vi "quiz 3.4.vi"() -> ()   [LabVIEW 2017]
panel:
  out "Tab Control":T1(tab)
  in  "Ingresar":bool
  in  "usuario":string
  in  "Contraseña":string
  in  "eliminar":bool
  in  "agregar":bool
  in  "Lista":bool
  in  "FINALIZAR":bool
  in  "Volver":bool
  in  "AÑADIR":bool
  in  "contraseña":string
  in  "usuario":string
  in  "Quitar":bool
  in  "usuario a eliminar":string
  in  "FINALIZAR 3":bool
  in  "Volver 2":bool
  out "Seccion Inicada por:":string
  in  "FINALIZAR 2":bool
  in  "FINALIZAR 4":bool
  in  "Volver 3":bool
  out "USUARIOS":string
  # "¿QUE DESEA REALIZAR?"
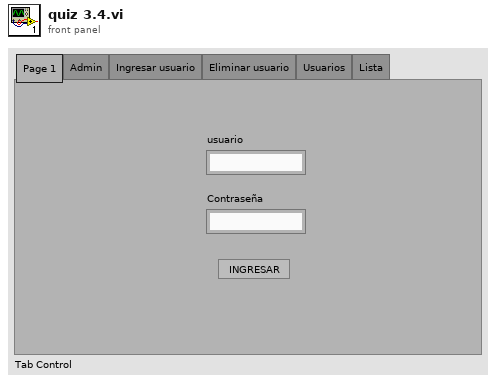
[diagram p1: front panel]
types:
  T1 = enum32{"Page 1", "Admin", "Ingresar usuario", "Eliminar usuario", "Usuarios", "Lista"}
  T2 = enum16{"open", "replace", "create", "open or create", "replace or create", "replace or create with confirmation"}
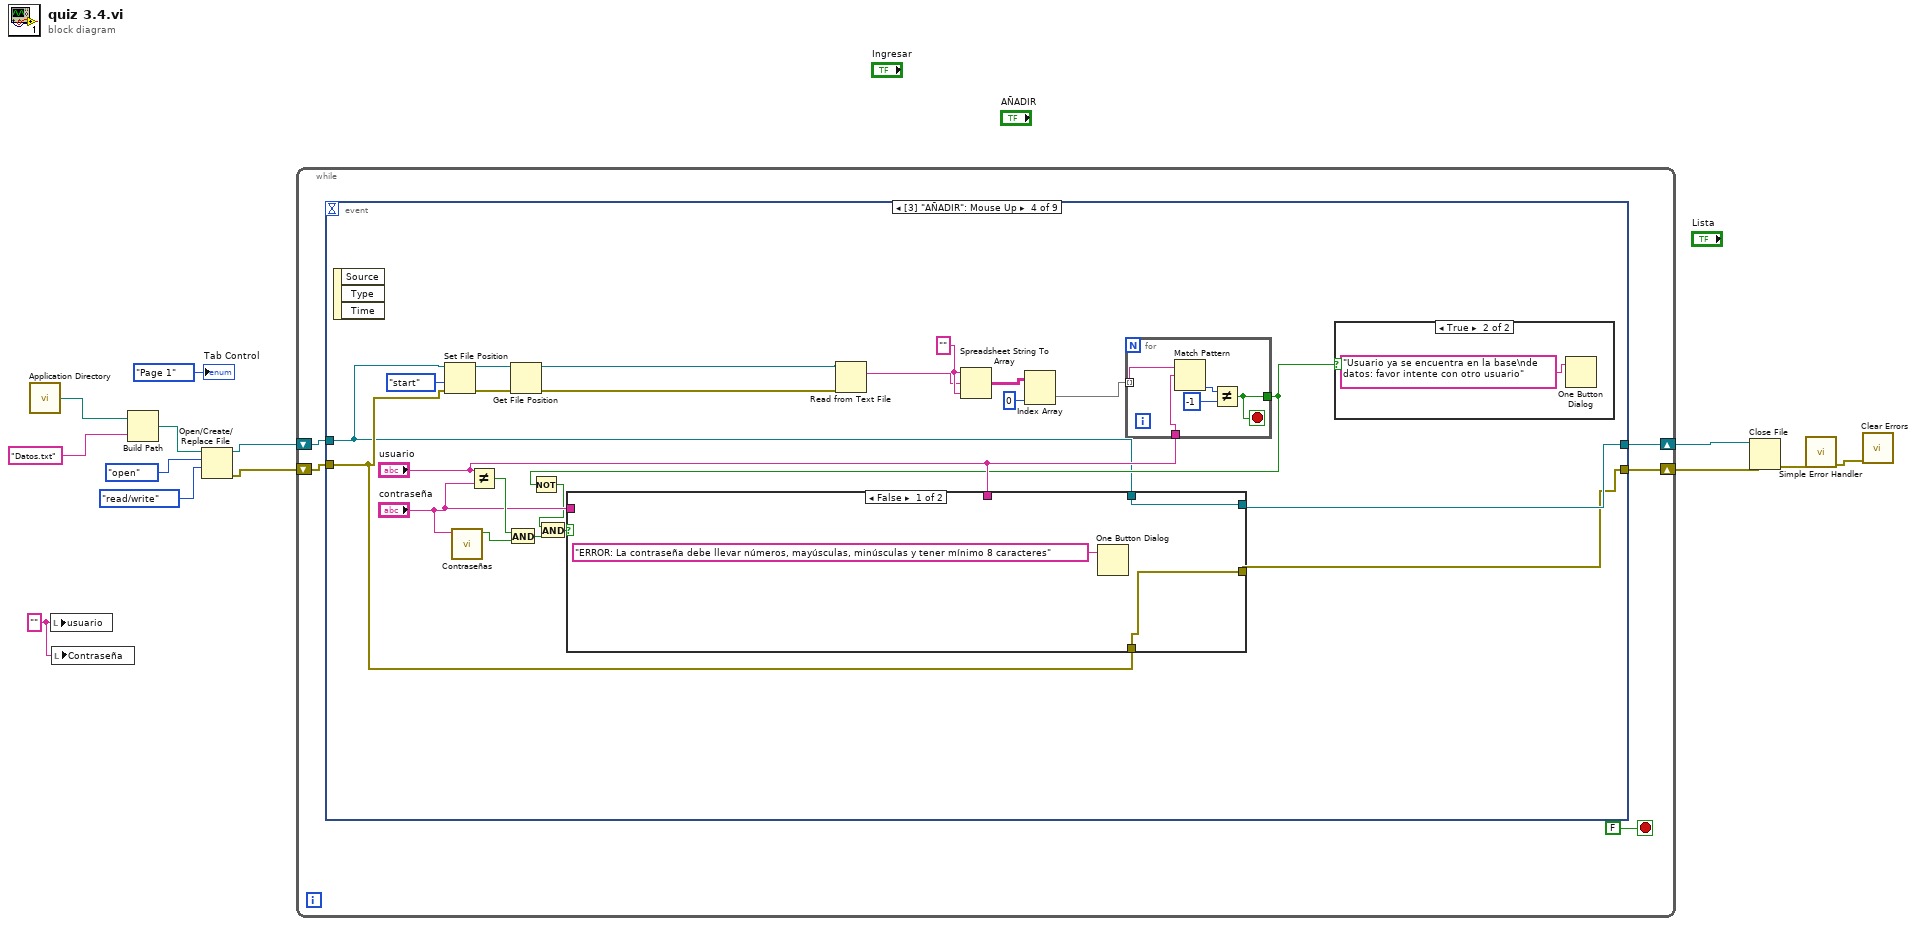
[diagram p0: block diagram]
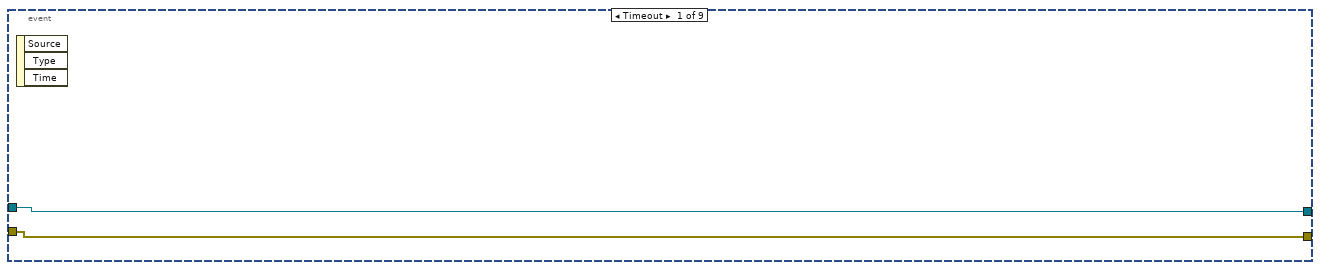
[diagram p2: hidden frame]
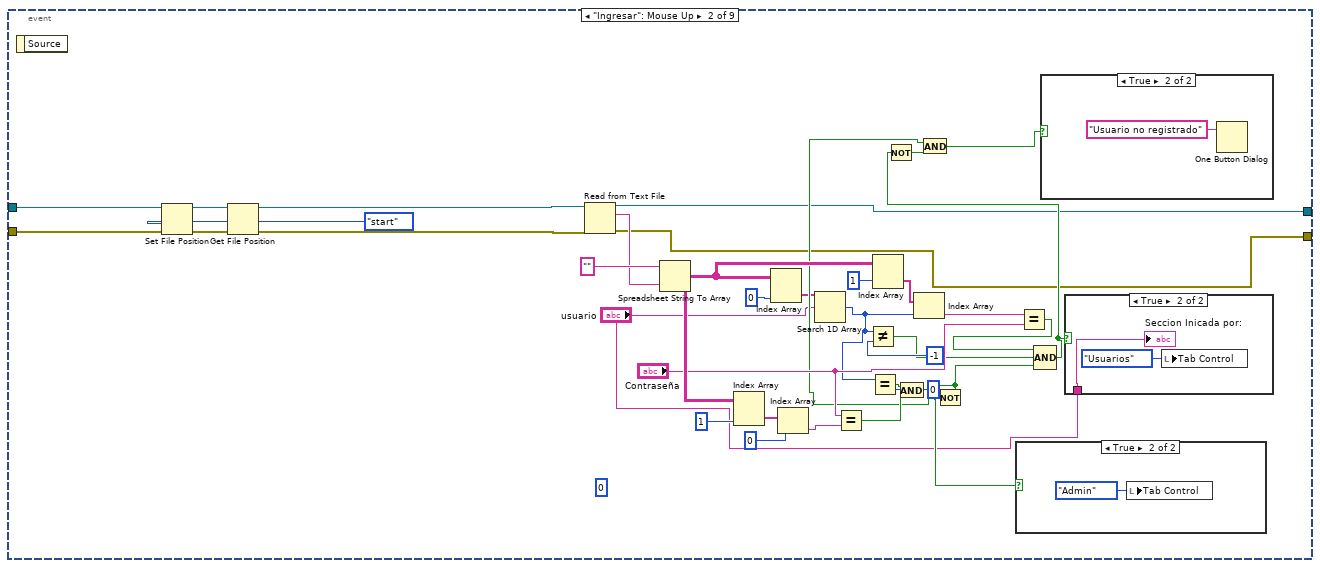
[diagram p3: hidden frame]
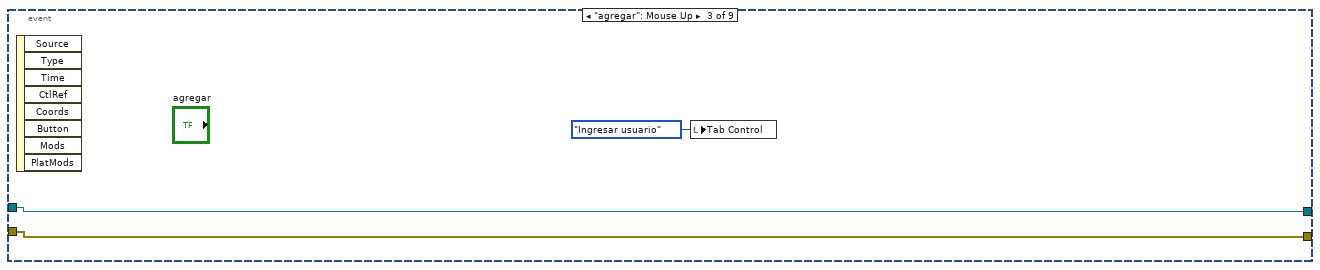
[diagram p7: hidden frame]
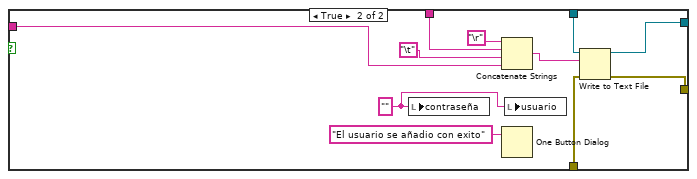
[diagram p9: hidden frame]
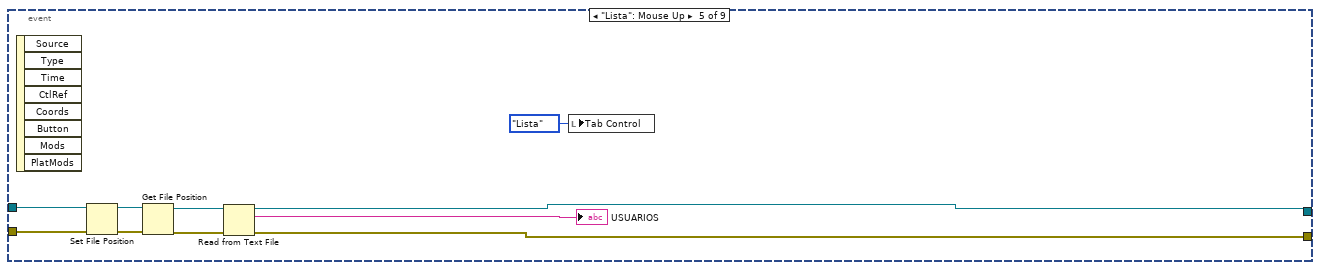
[diagram p10: hidden frame]
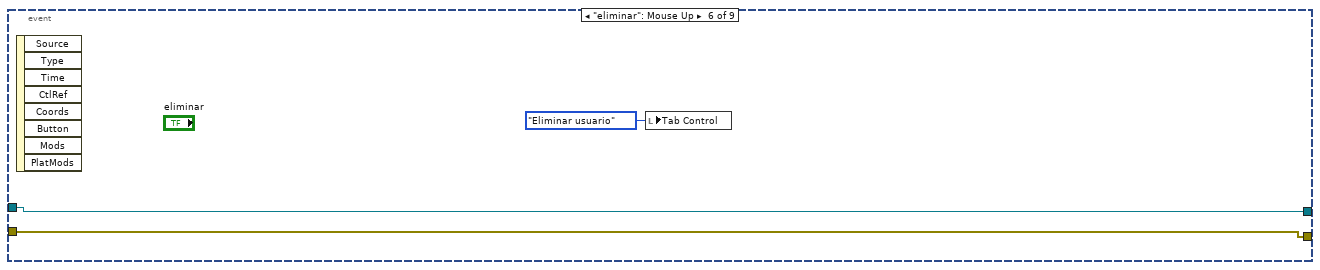
[diagram p11: hidden frame]
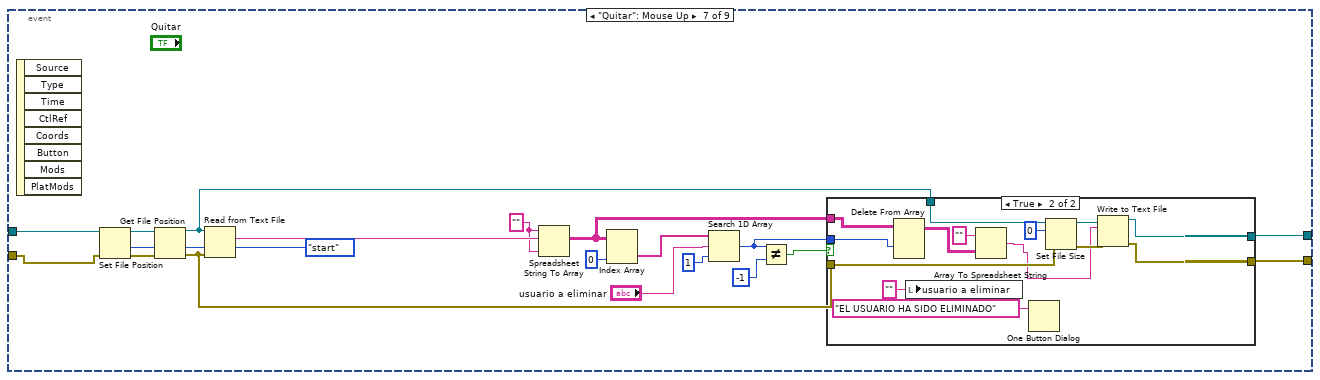
[diagram p12: hidden frame]
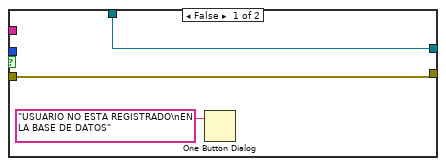
[diagram p13: hidden frame]
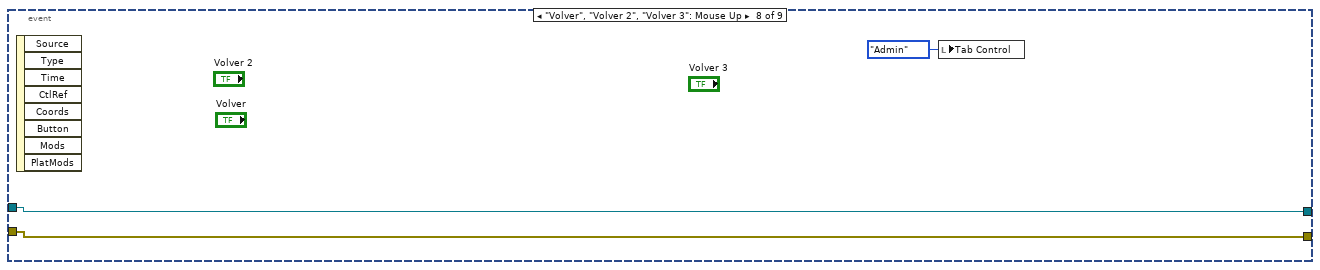
[diagram p14: hidden frame]
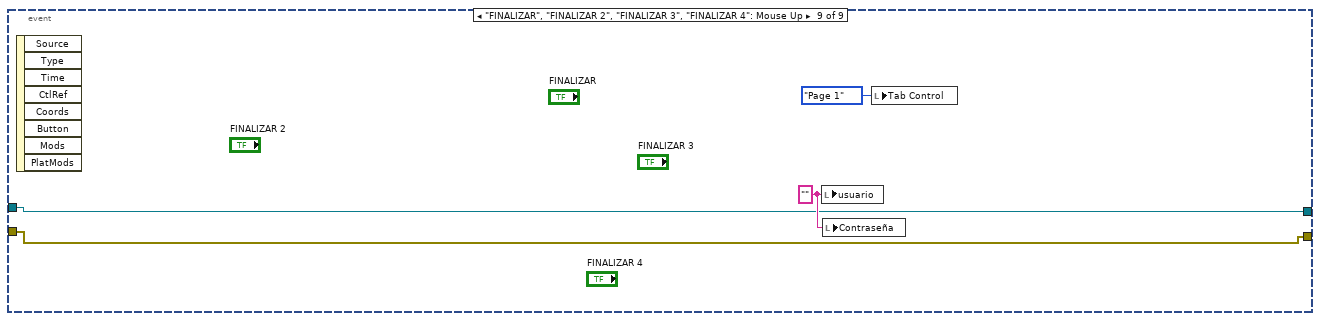
[diagram p15: hidden frame]
diagram:
  w2 = "" ("usuario")
  n1 = call <vilib>:"Application Directory.vi"() -> ("Application Directory"=w10:path)
  n2 = local write "usuario"(w2) -> ()
  n3 = local write "Contraseña"(w2) -> ()
  n4 = Build Path(base path=w10, name or relative path="Datos.txt") -> (appended path=w7:path)
  n5 = Open/Create/Replace File(file path (use dialog)=w7, operation (0:open)=T2."open", access (0:read/write)=enum16{"read/write", "read-only", "write-only"}."read/write") -> (refnum out=w8:refnum<file>, error out=w5:errorcluster)  [unwired: 3 in, 1 out]
  n6 = while {
    shift-right: [w14] -> w11
    shift-left: w8 -> [w16]
    shift-right: [w15] -> w6
    shift-left: w5 -> [w17]
    stop <- FALSE stop-if-true
    n7 = event shown="[3] \"AÑADIR\": Mouse Up" {
      selector: _ -> [_ _ _ _ _ _ _ _ _]
      dyn-events: _ -> [_ _ _ _ _ _ _ _ _]
      timeout: _ -> [_ _ _ _ _ _ _ _ _]
      tunnel: w16 -> [w20 w51 w62 w63 w112 w116 w133 w156 w159]
      tunnel: [w20 w24 w62 w81 w107 w116 w119 w156 w159] -> w14
      tunnel: w17 -> [w19 w47 w61 w64 w111 w117 w132 w155 w158]
      tunnel: [w19 w25 w61 w65 w106 w117 w120 w155 w158] -> w15
      event Timeout {
        n8 = event-data() -> ()  [unwired: 1 in, 3 out]
      }
      event "Ingresar": Mouse Up {
        (unwired) 0 ("index")
        n9 = event-data() -> ()  [unwired: 1 in, 1 out]
        n10 = Set File Position(refnum=w51, from (0:start)=enum16{"start", "end", "current"}."start", error in=w47) -> (refnum out=w55:refnum<file>, error out=w53:errorcluster)  [unwired: 1 in]
        n11 = Get File Position(4:w53, 7:w55) -> (0:w52:errorcluster, 3:w54:refnum<file>)  [unwired: 1 out]
        n12 = Read from Text File(file (use dialog)=w54, error in=w52) -> (refnum out=w24:refnum<file>, text=w49:string, error out=w25:errorcluster)  [unwired: 2 in, 1 out]
        n13 = Spreadsheet String To Array(format string="", spreadsheet string=w49, array type (2D Dbl)=w49) -> (array=w36:string[][])  [unwired: 1 in]
        n14 = Index Array(array=w36, index (col)=1 ("disabled index (col)")) -> (element=w41:string[])  [unwired: 1 in]
        n15 = Index Array(array=w36, index (col)=0 ("disabled index (col)")) -> (element=w23:string[])  [unwired: 1 in]
        n16 = Index Array(array=w41, index=0) -> (element=w39:string)
        n17 = Search 1D Array(1D array=w23, element="usuario") -> (index of element=w21:i32)  [unwired: 1 in]
        n18 = Equal?(x="Contraseña", y=w39) -> (x = y?=w38:bool)
        n19 = Not Equal?(x=w21, y=-1) -> (x != y?=w30:bool)
        n20 = Equal?(x=w21, y=0) -> (x = y?=w43:bool)
        n21 = Index Array(array=w36, index (col)=1 ("disabled index (col)")) -> (element=w34:string[])  [unwired: 1 in]
        n22 = And(x=w43, y=w38) -> (x .and. y?=w37:bool)
        n23 = Index Array(array=w34, index=w21) -> (element=w33:string)
        n24 = Not(x=w37) -> (.not. x?=w26:bool)
        n25 = case shown="True" w37 {
          frame False {
          }
          frame True {
            n26 = local write "Tab Control"(T1."Admin" ("Tab Control")) -> ()
          }
        }
        n27 = Equal?(x=w33, y="Contraseña") -> (x = y?=w31:bool)
        n28 = Compound Arithmetic op=AND(w31, w30, w26) -> (w28:bool)
        n29 = Not(x=w28) -> (.not. x?=w29:bool)
        n30 = And(x=w26, y=w29) -> (x .and. y?=w27:bool)
        n31 = case shown="True" w27 {
          frame False {
          }
          frame True {
            n32 = One Button Dialog(message="Usuario no registrado") -> ()  [unwired: 1 in, 1 out]
          }
        }
        n33 = case shown="True" w28 {
          tunnel: "usuario" -> [_ w58]
          frame False {
          }
          frame True {
            n34 = local write "Tab Control"(T1."Usuarios" ("Tab Control")) -> ()
            "Seccion Inicada por:" <- w58
          }
        }
      }
      event "agregar": Mouse Up {
        n35 = event-data() -> ()  [unwired: 1 in, 8 out]
        n36 = local write "Tab Control"(T1."Ingresar usuario" ("Tab Control")) -> ()
      }
      event "AÑADIR": Mouse Up {
        w75 = "" ("format string")
        n37 = event-data() -> ()  [unwired: 1 in, 3 out]
        n38 = Set File Position(refnum=w63, from (0:start)=enum16{"start", "end", "current"}."start", error in=w64) -> (refnum out=w80:refnum<file>, error out=w77:errorcluster)  [unwired: 1 in]
        n39 = call "Contraseñas.vi"("String"="contraseña") -> ("Contraseña Correcta?"=w84:bool)  [unwired: 10 in]
        n40 = Not Equal?(x="usuario", y="contraseña") -> (x != y?=w83:bool)
        n41 = And(x=w83, y=w84) -> (x .and. y?=w69:bool)
        n42 = Get File Position(4:w77, 7:w80) -> (0:w76:errorcluster, 3:w79:refnum<file>)  [unwired: 1 out]
        n43 = Read from Text File(file (use dialog)=w79, error in=w76) -> (text=w74:string)  [unwired: 2 in, 3 out]
        n44 = Spreadsheet String To Array(format string=w75, spreadsheet string=w74, array type (2D Dbl)=w75) -> (array=w73:string[][])  [unwired: 1 in]
        n45 = Index Array(array=w73, index (col)=0 ("disabled index (col)")) -> (element=w71:string[])  [unwired: 1 in]
        n46 = for {
          tunnel: w71 -> [w90] mode=indexing
          tunnel: "usuario" -> [w89]
          tunnel: [w86] -> w67
          stop <- w86 stop-if-true
          n47 = Match Pattern(string=w90, regular expression=w89) -> (offset past match=w88:i32)  [unwired: 1 in, 3 out]
          n48 = Not Equal?(x=w88, y=-1) -> (x != y?=w86:bool)
        }
        n49 = Not(x=w67) -> (.not. x?=w66:bool)
        n50 = And(x=w66, y=w69) -> (x .and. y?=w68:bool)
        n51 = case shown="False" w68 {
          tunnel: [w93 w104] -> w65
          tunnel: [w92 w103] -> w81
          tunnel: "usuario" -> [_ w102]
          tunnel: "contraseña" -> [_ w101]
          tunnel: w64 -> [w93 w96]
          tunnel: w63 -> [w92 w95]
          frame False {
            n52 = One Button Dialog(message="ERROR: La contraseña debe llevar números, mayúsculas, minúsculas y tener mínimo 8 caracteres") -> ()  [unwired: 1 in, 1 out]
          }
          frame True {
            w97 = "" ("contraseña")
            n53 = local write "contraseña"(w97) -> ()
            n54 = Concatenate Strings("\r", w102, "\t", w101) -> (w100:string)
            n55 = One Button Dialog(message="El usuario se añadio con exito") -> ()  [unwired: 1 in, 1 out]
            n56 = local write "usuario"(w97) -> ()
            n57 = Write to Text File(file (use dialog)=w95, text=w100, error in=w96) -> (refnum out=w103:refnum<file>, error out=w104:errorcluster)  [unwired: 1 in, 1 out]
          }
        }
        n58 = case shown="True" w67 {
          frame False {
          }
          frame True {
            n59 = One Button Dialog(message="Usuario ya se encuentra en la base\nde datos: favor intente con otro usuario") -> ()  [unwired: 1 in, 1 out]
          }
        }
      }
      event "Lista": Mouse Up {
        n60 = event-data() -> ()  [unwired: 1 in, 8 out]
        n61 = Set File Position(refnum=w112, error in=w111) -> (refnum out=w113:refnum<file>, error out=w114:errorcluster)  [unwired: 2 in]
        n62 = Get File Position(4:w114, 7:w113) -> (0:w109:errorcluster, 3:w110:refnum<file>)  [unwired: 1 out]
        n63 = Read from Text File(file (use dialog)=w110, error in=w109) -> (refnum out=w107:refnum<file>, text=→"USUARIOS":string, error out=w106:errorcluster)  [unwired: 2 in, 1 out]
        n64 = local write "Tab Control"(T1."Lista" ("Tab Control")) -> ()
      }
      event "eliminar": Mouse Up {
        n65 = event-data() -> ()  [unwired: 1 in, 8 out]
        n66 = local write "Tab Control"(T1."Eliminar usuario" ("Tab Control")) -> ()
      }
      event "Quitar": Mouse Up {
        w130 = "" ("format string")
        n67 = event-data() -> ()  [unwired: 1 in, 8 out]
        n68 = Set File Position(refnum=w133, from (0:start)=enum16{"start", "end", "current"}."start", error in=w132) -> (refnum out=w135:refnum<file>, error out=w136:errorcluster)  [unwired: 1 in]
        n69 = Get File Position(4:w136, 7:w135) -> (0:w121:errorcluster, 3:w122:refnum<file>)  [unwired: 1 out]
        n70 = Read from Text File(file (use dialog)=w122, error in=w121) -> (text=w131:string)  [unwired: 2 in, 3 out]
        n71 = Spreadsheet String To Array(format string=w130, spreadsheet string=w131, array type (2D Dbl)=w130) -> (array=w118:string[][])  [unwired: 1 in]
        n72 = Index Array(array=w118, index (col)=0 ("disabled index (col)")) -> (element=w124:string[])  [unwired: 1 in]
        n73 = Search 1D Array(1D array=w124, element="usuario a eliminar", start index (0)=1) -> (index of element=w123:i32)
        n74 = Not Equal?(x=w123, y=-1) -> (x != y?=w125:bool)
        n75 = case shown="True" w125 {
          tunnel: w123 -> [_ w143]
          tunnel: w122 -> [w139 w149]
          tunnel: w121 -> [w138 w148]
          tunnel: [w138 w153] -> w120
          tunnel: [w139 w152] -> w119
          tunnel: w118 -> [_ w144]
          frame False {
            n76 = One Button Dialog(message="USUARIO NO ESTA REGISTRADO\nEN LA BASE DE DATOS") -> ()  [unwired: 1 in, 1 out]
          }
          frame True {
            n77 = Delete From Array(array=w144, index (row)=w143) -> (array with subset deleted=w141:string[][])  [unwired: 2 in, 1 out]
            n78 = local write "usuario a eliminar"("" ("usuario a eliminar")) -> ()
            n79 = Array To Spreadsheet String(array=w141, 3:"" ("format string")) -> (spreadsheet string=w140:string)  [unwired: 1 in]
            n80 = One Button Dialog(message="EL USUARIO HA SIDO ELIMINADO") -> ()  [unwired: 1 in, 1 out]
            n81 = Set File Size(4:w148, 6:i64 0 ("size (in bytes)"), 7:w149) -> (0:w147:errorcluster, 3:w146:refnum<file>)
            n82 = Write to Text File(file (use dialog)=w146, text=w140, error in=w147) -> (refnum out=w152:refnum<file>, error out=w153:errorcluster)  [unwired: 1 in, 1 out]
          }
        }
      }
      event "Volver", "Volver 2", "Volver 3": Mouse Up {
        n83 = event-data() -> ()  [unwired: 1 in, 8 out]
        n84 = local write "Tab Control"(T1."Admin" ("Tab Control")) -> ()
      }
      event "FINALIZAR", "FINALIZAR 2", "FINALIZAR 3", "FINALIZAR 4": Mouse Up {
        w160 = "" ("usuario")
        n85 = event-data() -> ()  [unwired: 1 in, 8 out]
        n86 = local write "usuario"(w160) -> ()
        n87 = local write "Contraseña"(w160) -> ()
        n88 = local write "Tab Control"(T1."Page 1" ("Tab Control")) -> ()
      }
    }
  }
  n89 = Close File(refnum=w11, error in=w6) -> (error out=w4:errorcluster)  [unwired: 1 out]
  n90 = call <vilib>:"Simple Error Handler.vi"("error in (no error)"=w4) -> ("error out"=w3:errorcluster)  [unwired: 4 in, 4 out]
  n91 = call <vilib>:"Clear Errors.vi"("error in (no error)"=w3) -> ()  [unwired: 5 in, 2 out]
  "Tab Control" <- T1."Page 1" ("Tab Control")
